vi "Counter - Read Encoder (Continuous Clock).vi"() -> ()   [LabVIEW 2017]
doc: "本范例演示用一个计数器输入和一个外部时钟实现对编码器测量到的角位置连续采样的方法。\n\n关于将信号连接至DAQ设备的方法，可参考设备文档。"
uses:
  <vilib>/Utility/error.llb/DialogType.ctl
  <vilib>/DAQmx/read.llb/DAQmx Read (Counter 1D DBL 1Chan NSamp).vi
  <vilib>/DAQmx/create/channels.llb/DAQmx Create Channel (CI-Position-Angular Encoder).vi
  <vilib>/DAQmx/configure/timing.llb/DAQmx Timing (Sample Clock).vi
  <vilib>/DAQmx/miscellaneous.llb/DAQmx Fill In Error Info.vi
  <resource>/objmgr/daqmx.rc
panel:
  in  "Z索引接线端":tag="PFI9"
  in  "启用Z索引":bool
  in  "脉冲每转":u32=24
  in  "B输入接线端":tag="PFI10"
  in  "输入接线端":tag="PFI8"
  in  "计数器":tag="Dev1/ctr0"
  in  "触发类型":enum32{"No Trigger", "Digital Arm Start"}(tab)
  in  "边沿":i32(ring)=10280 items=["上升"=10280, "下降"=10171]
  in  "数字触发源":tag
  out "采集数据":dbl[](array[numeric])
  in  "停止":bool
  in  "每次循环采样数":i32=100
  in  "采样率":dbl=1000.0
  in  "采样时钟源":tag="PFI0"
  # "通道设置"
  # "采集数据"
  # "定时设置"
  # "触发设置"
  # "如需配置并使用触发/计数重置，必须先在上面选择相应的选项卡。  有些硬件不支持上述选项－更多信息见设备的相应文档。"
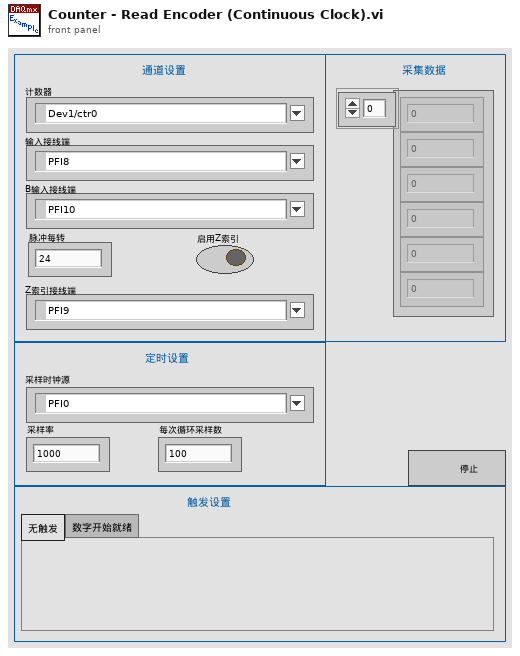
[diagram p1: front panel]
types:
  T1 = typedef "DialogType.ctl" = u16
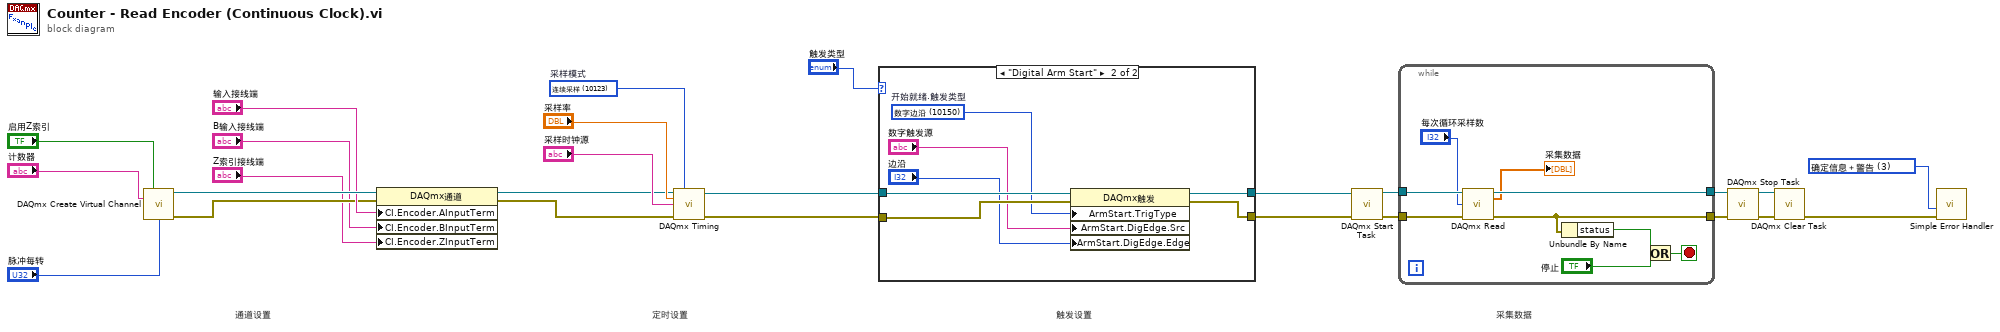
[diagram p0: block diagram]
diagram:
  w1 = T1 3 items=["无对话框", "确定信息", "继续或停止信息", "确定信息＋警告", "继续/停止＋警告"] ("对话框类型（确定信息：1）")
  w26 = 10123 items=["有限采样"=10178, "连续采样"=10123, "硬件定时单点"=12522]  # 采样模式
  # "采集数据"
  # "触发设置"
  # "定时设置"
  # "通道设置"
  n1 = call-poly <vilib>:"DAQmx Create Virtual Channel.vi"("z index enable"="启用Z索引", "counter"="计数器", "pulses per revolution"="脉冲每转") -> ("task out"=w14:refnum<k21>, "error out"=w12:errorcluster)  [unwired: 11 in]
  n2 = property class="DAQmx通道"(reference=w14, error in=w12, "CI.Encoder.AInputTerm"="输入接线端", "CI.Encoder.BInputTerm"="B输入接线端", "CI.Encoder.ZInputTerm"="Z索引接线端") -> (reference out=w8:refnum<k21>, error out=w7:errorcluster)
  n3 = call-poly <vilib>:"DAQmx Timing.vi"("task/channels in"=w8, "sample mode"=w26, "rate"="采样率", "source"="采样时钟源", "error in"=w7) -> ("task out"=w17:refnum<k21>, "error out"=w16:errorcluster)  [unwired: 9 in]
  n4 = case shown="\"Digital Arm Start\"" "触发类型" {
    tunnel: w17 -> [w28 w35]
    tunnel: w16 -> [w27 w32]
    tunnel: [w28 w34] -> w18
    tunnel: [w27 w33] -> w19
    frame "No Trigger", Default {
    }
    frame "Digital Arm Start" {
      w29 = 10150 items=["数字边沿"=10150, "无"=10230]  # 开始就绪.触发类型
      n5 = property class="DAQmx触发"(reference=w35, error in=w32, "ArmStart.TrigType"=w29, "ArmStart.DigEdge.Src"="数字触发源", "ArmStart.DigEdge.Edge"="边沿") -> (reference out=w34:refnum<k21>, error out=w33:errorcluster)
    }
  }
  n6 = call <vilib>:"DAQmx Start Task.vi"("task/channels in"=w18, "error in"=w19) -> ("task out"=w25:refnum<k21>, "error out"=w24:errorcluster)  [unwired: 12 in]
  n7 = while {
    tunnel: w25 -> [w44]
    tunnel: w24 -> [w43]
    tunnel: [w40] -> w4
    tunnel: [w41] -> w5
    stop <- w42 stop-if-true
    n8 = call-poly <vilib>:"DAQmx Read.vi"("task/channels in"=w44, "number of samples per channel"="每次循环采样数", "error in"=w43) -> ("task out"=w41:refnum<k21>, "data"=→"采集数据":dbl[], "error out"=w40:errorcluster)  [unwired: 10 in]
    n9 = Unbundle By Name(w40) -> ("status"=w39:bool)
    n10 = Or(x=w39, y="停止") -> (x .or. y?=w42:bool)
  }
  n11 = call <vilib>:"DAQmx Stop Task.vi"("task/channels in"=w5, "error in"=w4) -> ("task out"=w2:refnum<k21>, "error out"=w3:errorcluster)  [unwired: 12 in]
  n12 = call <vilib>:"DAQmx Clear Task.vi"("task in"=w2, "error in"=w3) -> ("error out"=w23:errorcluster)  [unwired: 13 in]
  n13 = call <vilib>:"Simple Error Handler.vi"("type of dialog (OK msg:1)"=w1, "error in (no error)"=w23) -> ()  [unwired: 3 in, 5 out]
